vi "RB Control.vi"(8 "error in":errorcluster, 10 "Channels":i32, 11 "Radio Ref":refnum<vi>) -> (0 "error out":errorcluster)   [LabVIEW 2025, in "DMM.lvlib" / "DMM Instrument.lvclass"]
uses:
  DMM Instrument.lvclass
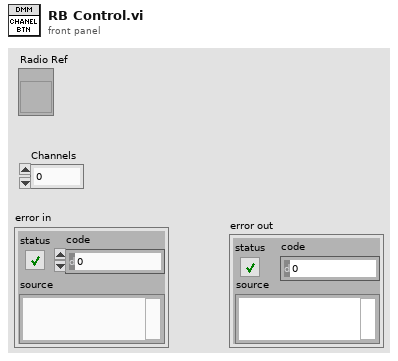
[diagram p1: front panel]
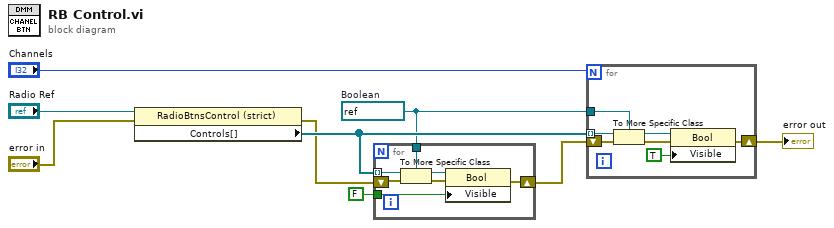
[diagram p0: block diagram]
diagram:
  w5 = refnum<vi> refnum  # Boolean
  n1 = property class="RadioBtnsControl (strict)"(reference="Radio Ref", error in="error in") -> (error out=w3:errorcluster, "Controls[]"=w7:refnum<vi>[])  [unwired: 1 out]
  n2 = for {
    tunnel: w7 -> [w15] mode=indexing
    tunnel: w5 -> [w14]
    tunnel: FALSE ("Visible") -> [w13]
    shift-right: [w10] -> w2
    shift-left: w3 -> [w12]
    n3 = To More Specific Class(target class=w14, reference=w15, error in=w12) -> (specific class reference=w16:refnum<vi>, error out=w11:errorcluster)
    n4 = property class="Bool"(reference=w16, error in=w11, "Visible"=w13) -> (error out=w10:errorcluster)  [unwired: 1 out]
  }
  n5 = for {
    N: "Channels" -> [_]
    tunnel: w7 -> [w22] mode=indexing
    tunnel: w5 -> [w21]
    shift-right: [w18] -> w1
    shift-left: w2 -> [w17]
    n6 = To More Specific Class(target class=w21, reference=w22, error in=w17) -> (specific class reference=w23:refnum<vi>, error out=w19:errorcluster)
    n7 = property class="Bool"(reference=w23, error in=w19, "Visible"=TRUE) -> (error out=w18:errorcluster)  [unwired: 1 out]
  }
  "error out" <- w1
